vi "Open TDMS File.vi"(7 "user event queue in":refnum<queue>, 8 "error in":errorcluster, 10 "file path":variant, 11 "class objects":T2) -> (0 "error out":errorcluster, 3 "class object":T2, 5 "user event queue out":refnum<queue>)   [LabVIEW 2011]
uses:
  Controls/Class Objects.ctl
  Modules/File/Configuration/Configuration.lvclass
  Modules/Hardware/Power Supply/Power Supply.lvclass
  Modules/Hardware/Mass Flow Controller/Mass Flow Controller.lvclass
  Modules/Hardware/PID/PID.lvclass
  Modules/Hardware/Valve Controller/Valve Controller.lvclass
  Modules/Hardware/Multimeter/Multimeter.lvclass
  Modules/Hardware/Vapour Generator/Vapour Generator.lvclass
  Modules/File/TDMS/TDMS.lvclass
  Controls/User Event Control.ctl
  Controls/User Event Action.ctl
  Functional Global Data/Globals.ctl
  Controls/User Interface Action.ctl
  Modules/Menu/Menu Action.ctl
  Controls/TDMS File Handling.ctl
  Controls/Class Labels.ctl
  Controls/Display Mode.ctl
panel:
  in  "OK":bool
  in  "Select Data Type":T1(radio)
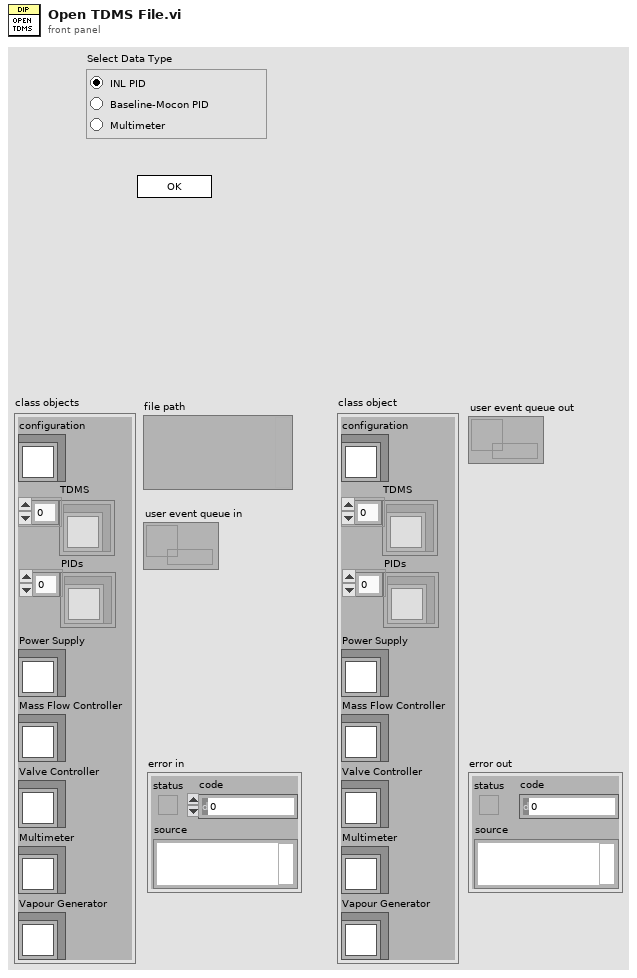
[diagram p1: front panel]
types:
  T1 = enum32{"INL PID", "Baseline-Mocon PID", "Multimeter"}
  T2 = typedef "Class Objects.ctl" = cluster{"configuration":refnum<class "Configuration.lvclass">, "TDMS":refnum<class "TDMS.lvclass">[], "Power Supply":refnum<class "Power Supply.lvclass">, "Mass Flow Controller":refnum<class "Mass Flow Controller.lvclass">, "Valve Controller":refnum<class "Valve Controller.lvclass">, "Multimeter":refnum<class "Multimeter.lvclass">, "Vapour Generator":refnum<class "Vapour Generator.lvclass">, "PIDs":refnum<class "PID.lvclass">[]}
  T3 = typedef "Globals.ctl" = enum16{"Initialize", "Get DAQ Params", "Get Data Display Params", "Set DAQ Params", "Set Data Display Params"}
  T4 = typedef "User Interface Action.ctl" = enum16{"Initialize", "Data Acquisition Disable", "Data View Disable", "Sample Set", "Sample Set 2D Data", "Sample Set x0 & dx", "Sample Add", "Sample Set Cursor", "Sample Set Offset & Multiplier", "Sample Set Axis Labels", "Sample Parameters Disabled", "Sample Parameters Update", "Run Update", "Run Set Offset & Multiplier", "Run Set Axis Labels", "Run Set Cursor", "Run Set Disabled", "Run Parameters Update", "Run Parameters Disabled", "Run Number Set", "Run Number Set Range", "Run Number Set Disabled", "Sample Number Set", "Sample Number Set Range", "Notes Set Value", "Update Plot", "Set Plot Parameters", "Update Concentration Plot", "Time Set", "Clear DAQ Display", "Clear Analysis Display", "Status Bar Set", "Progress Bar Set", "Display Mode Set", "Experiment Type Set", "Analysis Plot Average Set", "Stop"}
  T5 = typedef "Menu Action.ctl" = enum16{"Initialize", "Insert Item", "Remove Item", "Set Checked Item", "Get Checked Item", "Get Item Index", "Item Present?", "Stop"}
  T6 = typedef "TDMS File Handling.ctl" = enum16{"Add TDMS File", "Get Active TDMS File", "Set Active TDMS File", "Set Active TDMS File Index"}
  T7 = typedef "Class Labels.ctl" = enum16{"Configuration", "TDMS", "PID", "Power Supply", "Vapour Generator", "MFC", "NMR", "Valve Controller", "Multimeter"}
  T8 = typedef "User Event Control.ctl" = cluster{"action":T9, "data":variant}
  T9 = typedef "User Event Action.ctl" = enum16{"Program Initialization", "Device Connections", "Device Settings", "Options", "DAQ Init", "PID Sample Test", "PID with PS Challenge", "PID with MFC Challenge", "Multimeter Sample Test", "Multimeter with MFC Challenge", "DAQ Stop", "Open Data File", "View Data File", "Change Display Mode", "Load INL PID Run Data", "Load Baseline-Mocon PID Data", "Load Multimeter Data", "Set Channel Sample", "Key Down", "Add Spectrum to Plot", "Add History to Plot", "Export History to Excel", "Clear Plots", "Save Plot", "Save Spectral Variable", "History Cursor Release", "Analysis Plot Cursor Release", "Program Deinitialization"}
  T10 = typedef "Display Mode.ctl" = enum16{"Sample", "Run"}
  T11 = typedef "Data Display Parameters.ctl" = cluster{"Number of Channels":u32, "Number of Groups":u32, "Display Mode":T10, "Data Type":string}
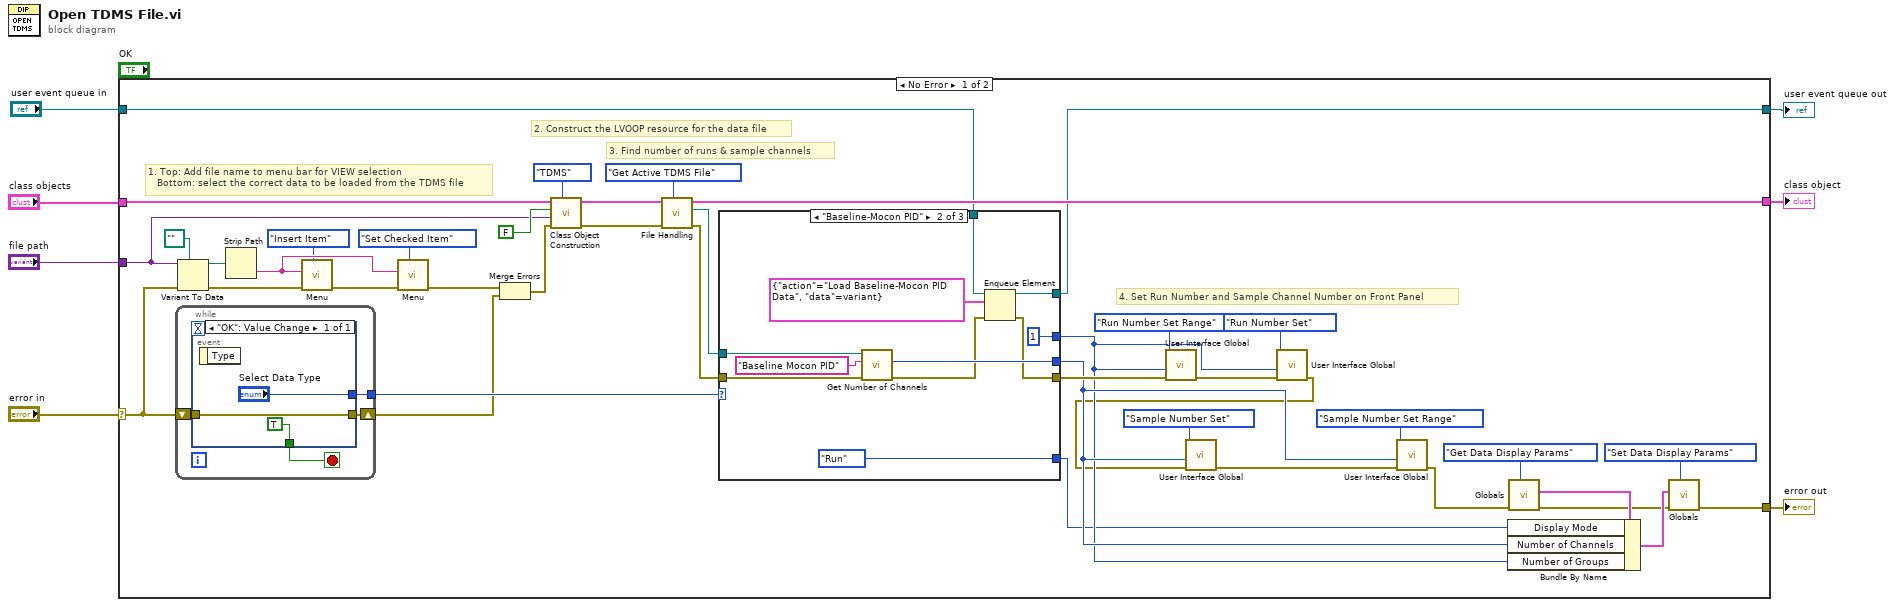
[diagram p0: block diagram]
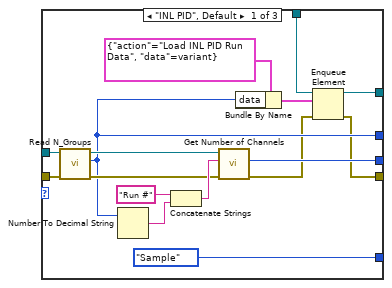
[diagram p2: hidden frame]
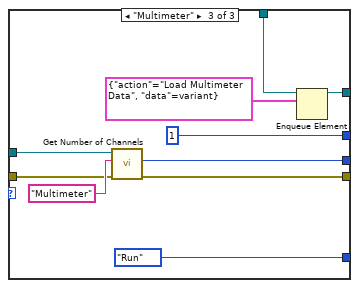
[diagram p3: hidden frame]
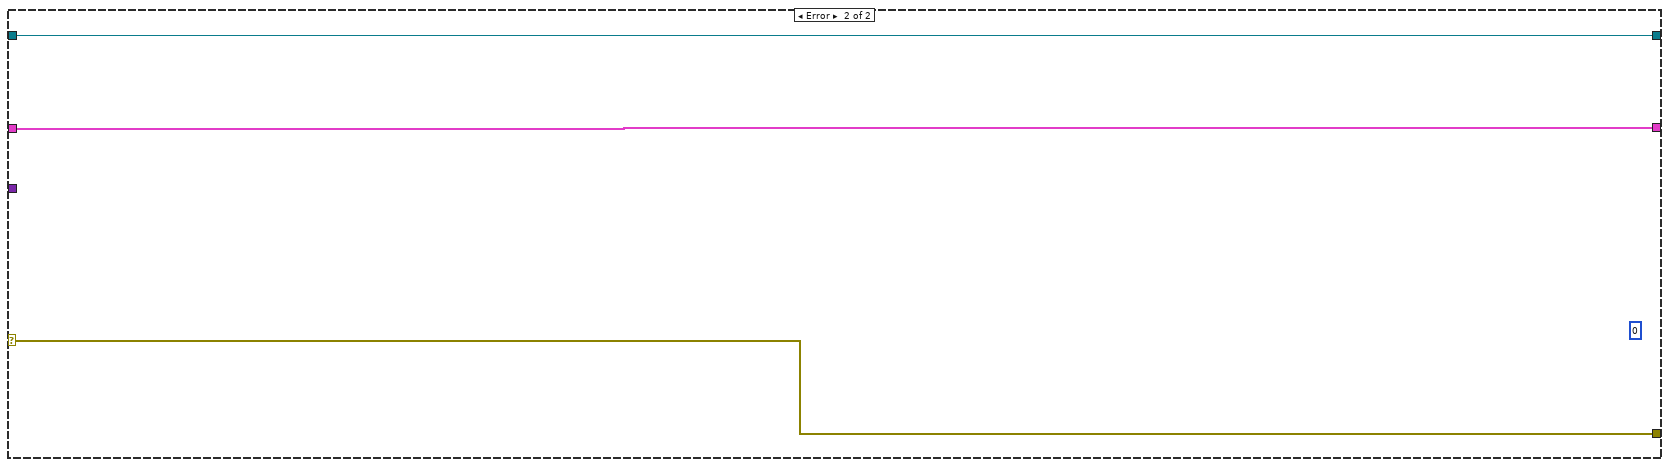
[diagram p4: hidden frame]
diagram:
  n1 = case shown="No Error" "error in" {
    selector: "error in" -> [w31 w95]
    tunnel: [w21 w95] -> w7
    tunnel: "file path" -> [w32 _]
    tunnel: [w39 w96] -> w6
    tunnel: "class objects" -> [w33 w96]
    tunnel: "user event queue in" -> [w15 w94]
    tunnel: [w14 w94] -> w1
    frame No Error {
      # "4. Set Run Number and Sample Channel Number on Front Panel"
      # "3. Find number of runs & sample channels"
      # "2. Construct the LVOOP resource for the data file"
      # "1. Top: Add file name to menu bar for VIEW selection\n   Bottom: select the correct data to be loaded from the TDMS file"
      n2 = while {
        tunnel: [w90] -> w17
        shift-right: [w88] -> w11
        shift-left: w31 -> [w89]
        stop <- w87 stop-if-true
        n3 = event shown="[0] \"OK\": Value Change" {
          selector: _ -> [_]
          dyn-events: _ -> [_]
          timeout: _ -> [_]
          tunnel: ["Select Data Type"] -> w90
          tunnel: w89 -> [w92]
          tunnel: [w92] -> w88
          tunnel: [TRUE] -> w87
          event "OK": Value Change {
            n4 = event-data() -> ()  [unwired: 1 in, 1 out]
          }
        }
      }
      n5 = Variant To Data(error in=w31, type=path "", Variant=w32) -> (data=w47:path, error out=w45:errorcluster)
      n6 = Strip Path(path=w47) -> (name=w44:string)  [unwired: 1 out]
      n7 = call "Menu.vi"("action"=Menu_Action."Insert Item" ("Menu"), "error in"=w45, "item tag"=w44) -> ("error out"=w46:errorcluster)  [unwired: 5 in, 3 out]
      n8 = call "Menu.vi"("action"=Menu_Action."Set Checked Item" ("Menu"), "error in"=w46, "item tag"=w44) -> ("error out"=w13:errorcluster)  [unwired: 5 in, 3 out]
      n9 = Merge Errors(w13, w11) -> (w12:errorcluster)
      n10 = call "Class Object Construction.vi"("class"=Class_Labels."TDMS" ("Class"), "error in"=w12, "param2"=w32, "param 1"=FALSE, "classes in"=w33) -> ("error out"=w37:errorcluster, "classes out"=w38:T2)  [unwired: 4 in]
      n11 = call "File Handling.vi"("TDMS File Handling"=TDMS_File_Handling."Get Active TDMS File", "error in"=w37, "Class objects"=w38) -> ("error out"=w27:errorcluster, "TDMS File"=w28:refnum<class "TDMS.lvclass">, "Class objects"=w39:T2)  [unwired: 6 in]
      n12 = case shown="\"Baseline-Mocon PID\"" w17 {
        tunnel: w28 -> [w65 w74 w85]
        tunnel: w27 -> [w64 w75 w84]
        tunnel: [w55 u16 1 ("N_Groups") u16 1 ("N_Groups")] -> w18
        tunnel: [w51 w66 w83] -> w23
        tunnel: [w61 w72 w82] -> w20
        tunnel: [Display_Mode."Sample" ("Display Mode") Display_Mode."Run" ("Display Mode") Display_Mode."Run" ("Display Mode")] -> w16
        tunnel: w15 -> [w53 w69 w79]
        tunnel: [w50 w68 w78] -> w14
        frame "INL PID", Default {
          n13 = call-dynamic "Read N_Groups.vi"("error in"=w64, "TDMS in"=w65) -> ("error out"=w58:errorcluster, "N_Groups"=w55:u16, "TDMS out"=w63:refnum<class "TDMS.lvclass">)  [unwired: 7 in]
          n14 = Number To Decimal String(number=w55) -> (decimal integer string=w59:string)  [unwired: 1 in]
          n15 = Concatenate Strings("Run #" ("Group Name"), w59) -> (w60:string)
          n16 = call-dynamic "Get Number of Channels.vi"("error in"=w58, "Group Name"=w60, "TDMS in"=w63) -> ("error out"=w52:errorcluster, "number of channels"=w61:i32)  [unwired: 6 in, 1 out]
          n17 = Bundle By Name(cluster=T8 {"action"=enum."Load INL PID Run Data", "data"=variant} ("element"), "data"=w55) -> (w54:T8)
          n18 = Enqueue Element(queue=w53, element=w54, error in (no error)=w52) -> (queue out=w50:refnum<queue>, error out=w51:errorcluster)  [unwired: 1 in, 1 out]
        }
        frame "Baseline-Mocon PID" {
          n19 = call-dynamic "Get Number of Channels.vi"("error in"=w75, "Group Name"="Baseline Mocon PID", "TDMS in"=w74) -> ("error out"=w67:errorcluster, "number of channels"=w72:i32)  [unwired: 6 in, 1 out]
          n20 = Enqueue Element(queue=w69, element=T8 {"action"=enum."Load Baseline-Mocon PID Data", "data"=variant}, error in (no error)=w67) -> (queue out=w68:refnum<queue>, error out=w66:errorcluster)  [unwired: 1 in, 1 out]
        }
        frame "Multimeter" {
          n21 = call-dynamic "Get Number of Channels.vi"("error in"=w84, "Group Name"="Multimeter", "TDMS in"=w85) -> ("error out"=w83:errorcluster, "number of channels"=w82:i32)  [unwired: 6 in, 1 out]
          n22 = Enqueue Element(queue=w79, element=T8 {"action"=enum."Load Multimeter Data", "data"=variant}) -> (queue out=w78:refnum<queue>)  [unwired: 2 in, 2 out]
        }
      }
      n23 = call "User Interface Global.vi"("error in"=w23, "data1"=w18, "action"=User_Interface_Action."Run Number Set Range") -> ("error out"=w49:errorcluster)  [unwired: 8 in]
      n24 = call "User Interface Global.vi"("error in"=w49, "data1"=w18, "action"=User_Interface_Action."Run Number Set") -> ("error out"=w8:errorcluster)  [unwired: 8 in]
      n25 = call "User Interface Global.vi"("error in"=w8, "data1"=w20, "action"=User_Interface_Action."Sample Number Set") -> ("error out"=w26:errorcluster)  [unwired: 8 in]
      n26 = call "User Interface Global.vi"("error in"=w26, "data1"=w20, "action"=User_Interface_Action."Sample Number Set Range") -> ("error out"=w10:errorcluster)  [unwired: 8 in]
      n27 = call "Globals.vi"("action"=Globals."Get Data Display Params", "error in"=w10) -> ("error out"=w9:errorcluster, "Data Display Params"=w29:T11)  [unwired: 7 in, 1 out]
      n28 = Bundle By Name(cluster=w29, "Display Mode"=w16, "Number of Channels"=w20, "Number of Groups"=w18) -> (w19:T11)
      n29 = call "Globals.vi"("action"=Globals."Set Data Display Params", "error in"=w9, "Data Display Params"=w19) -> ("error out"=w21:errorcluster)  [unwired: 6 in, 2 out]
    }
    frame Error {
      (unwired) u16 0 ("N_Groups")
    }
  }
  "error out" <- w7
  "class object" <- w6
  "user event queue out" <- w1
